vi "G Cluster to PLC Byte Stream.vi"(6 "Byte Length":i32, 8 "error in (no error)":errorcluster, 9 "[Sub-Item Type Descriptor]":T1[](array[typedef]), 10 "Value":variant, 11 "TwinCAT ADS in":refnum<class "TwinCAT ADS.lvclass">) -> (0 "error out":errorcluster, 2 "Byte Stream":u8[](array[numeric]), 3 "TwinCAT ADS out":refnum<class "TwinCAT ADS.lvclass">)   [LabVIEW 2018, in "TwinCAT ADS.lvclass"]
uses:
  TwinCAT ADS.lvclass
  Controls/PLC Sub-Item Type Descriptor.ctl
  Controls/PLC Type.ctl
  G Primitive to PLC Byte Stream.vi/ebfc1059-5ad7-41af-9a32-6ba056cec1e2.vi
  G Primitive to PLC Byte Stream.vi/6e01a951-886b-41b5-8cd1-fdd71fd1a533.vi
  G Primitive to PLC Byte Stream.vi/09c7a0ef-3209-4624-b801-f77696e71225.vi
  G Primitive to PLC Byte Stream.vi/97b8602c-6a72-408e-90bf-08a26de32539.vi
  G Primitive to PLC Byte Stream.vi/0fd4fbf3-4a18-432c-8f70-6a5c8fef8454.vi
  G Primitive to PLC Byte Stream.vi/afdb5a5e-237c-4be5-828e-15f510cf6cea.vi
  G Primitive to PLC Byte Stream.vi/185a6e12-4d7d-4ad7-9936-0525adb2f85e.vi
  G Primitive to PLC Byte Stream.vi/88229fb8-b58c-494b-bd2b-fea6e0d0ed1b.vi
  G Primitive to PLC Byte Stream.vi/e57df404-389c-41d0-a67c-37c75754ab31.vi
  G Primitive to PLC Byte Stream.vi/d0ee652c-9b86-46ed-9065-57d03aa8de3e.vi
  G Primitive to PLC Byte Stream.vi/886bf0b9-f01c-4a44-b2e2-abccc7b97bfa.vi
  G Primitive to PLC Byte Stream.vi/35f71df7-fc14-4c4d-983c-cf72c138dc9e.vi
  G Primitive to PLC Byte Stream.vi/2d2bc992-a9ff-4dd8-b8fe-74c21cb85899.vi
  G Primitive to PLC Byte Stream.vi/100e4a11-5e4a-45b7-be98-adc9eaebd48d.vi
  G Primitive to PLC Byte Stream.vi/132946d9-68c7-4ade-a66d-dc369520c644.vi
  <vilib>/Utility/error.llb/Trim Whitespace.vi
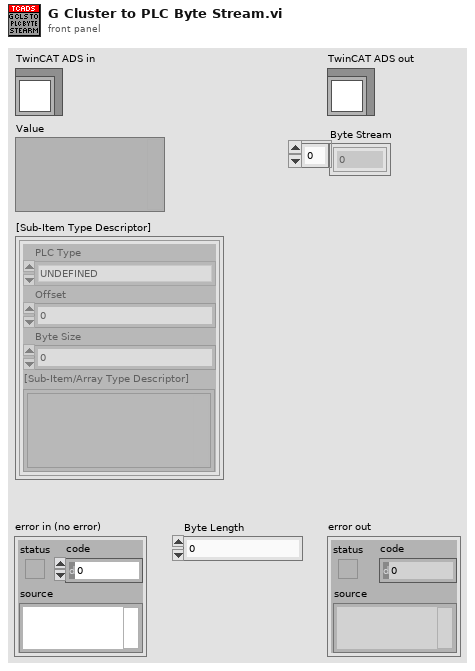
[diagram p1: front panel]
types:
  T1 = typedef "TwinCAT ADS.lvclass/PLC Sub-Item Type Descriptor.ctl" = cluster{"PLC Type":T2, "Offset":i32, "Byte Size":i32, "[Sub-Item/Array Type Descriptor]":variant[]}
  T2 = typedef "TwinCAT ADS.lvclass/PLC Type.ctl" = enum16{"UNDEFINED", "INT", "DINT", "REAL", "LREAL", "SINT", "BYTE", "UINT", "UDINT", "LINT", "ULINT", "STRING", "WSTRING", "BOOL", "TIME", "LTIME", "DATE", "DT", "TOD", "ARRAY", "JAGGED ARRAY", "STRUCT", "FUNCTION BLOCK", "UNION", "POINTER", "USER DEFINED"}
  T3 = typedef "TwinCAT ADS.lvclass/PLC Array Type Descriptor.ctl" = cluster{"Fundamental PLC Type":T2, "Fundamental Type Byte Size":i32, "Item Count":i32, "Dimension Lengths":i32[], "Sub-Item Type Descriptor":variant}
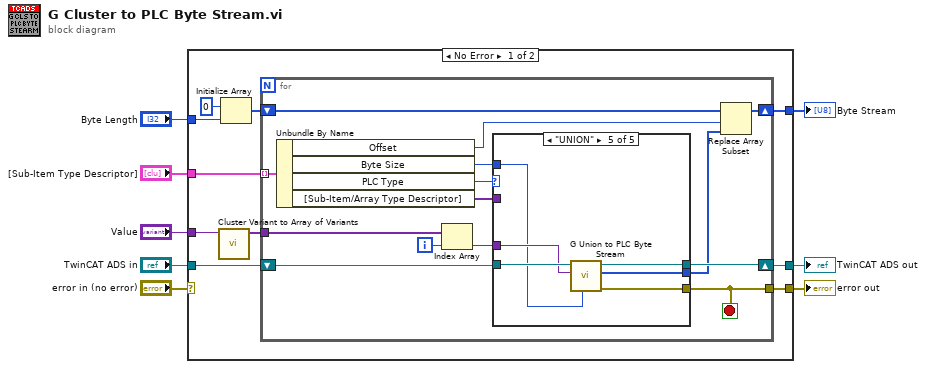
[diagram p0: block diagram]
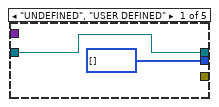
[diagram p2: hidden frame]
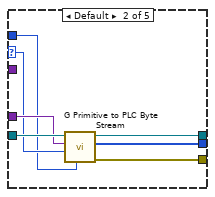
[diagram p3: hidden frame]
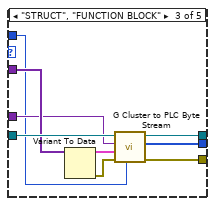
[diagram p4: hidden frame]
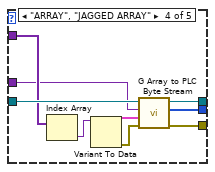
[diagram p5: hidden frame]
diagram:
  n1 = case shown="No Error" "error in (no error)" {
    selector: "error in (no error)" -> [_ w66]
    tunnel: "TwinCAT ADS in" -> [w18 w67]
    tunnel: [w17 w67] -> w7
    tunnel: "[Sub-Item Type Descriptor]" -> [w16 _]
    tunnel: "Value" -> [w15 _]
    tunnel: "Byte Length" -> [w14 _]
    tunnel: [w13 w66] -> w3
    tunnel: [w12 _] -> w2
    frame No Error {
      n2 = call "Cluster Variant to Array of Variants.vi"("Cluster Variant"=w15) -> ("[Variant]"=w11:variant[])  [unwired: 9 in, 1 out]
      n3 = Initialize Array(u8 0 ("Offset"), w14) -> (w9:u8[])
      n4 = for {
        shift-right: [w31] -> w17
        shift-left: w18 -> [w32]
        tunnel: w16 -> [w30] mode=indexing
        tunnel: w11 -> [w29]
        shift-right: [w23] -> w12
        shift-left: w9 -> [w24]
        tunnel: [w27] -> w13
        i -> [w28]
        stop <- w27 stop-if-true
        n5 = Unbundle By Name(w30) -> ("Offset"=w20:i32, "Byte Size"=w21:i32, "PLC Type"=w26:T2, "[Sub-Item/Array Type Descriptor]"=w25:variant[])
        n6 = Index Array(array=w29, index=w28) -> (element=w19:variant)
        n7 = case shown="\"UNION\"" w26 {
          selector: w26 -> [_ w37 _ _ _]
          tunnel: w32 -> [w34 w41 w50 w59 w65]
          tunnel: [w34 w39 w49 w52 w63] -> w31
          tunnel: [_ w40 w48 w53 w64] -> w27
          tunnel: w25 -> [_ _ w47 w58 _]
          tunnel: w19 -> [_ w38 w44 w56 w61]
          tunnel: [u8[] [] ("initialized array") w36 w43 w51 w62] -> w22
          tunnel: w21 -> [_ w35 w42 _ w60]
          frame "UNDEFINED", "USER DEFINED" {
          }
          frame Default {
            n8 = call "G Primitive to PLC Byte Stream.vi"("Byte Length"=w35, "PLC Type"=w37, "Value"=w38, "TwinCAT ADS in"=w41) -> ("error out"=w40:errorcluster, "Byte Stream"=w36:u8[], "TwinCAT ADS out"=w39:refnum<class "TwinCAT ADS.lvclass">)  [unwired: 5 in]
          }
          frame "STRUCT", "FUNCTION BLOCK" {
            n9 = Variant To Data(Variant=w47) -> (data=w45:T1[], error out=w46:errorcluster)  [unwired: 2 in]
            n10 = call "G Cluster to PLC Byte Stream.vi"("Byte Length"=w42, "error in (no error)"=w46, "[Sub-Item Type Descriptor]"=w45, "Value"=w44, "TwinCAT ADS in"=w50) -> ("error out"=w48:errorcluster, "Byte Stream"=w43:u8[], "TwinCAT ADS out"=w49:refnum<class "TwinCAT ADS.lvclass">)  [unwired: 4 in]
          }
          frame "ARRAY", "JAGGED ARRAY" {
            n11 = Index Array(array=w58) -> (element=w57:variant)  [unwired: 1 in]
            n12 = Variant To Data(Variant=w57) -> (data=w54:T3, error out=w55:errorcluster)  [unwired: 2 in]
            n13 = call "G Array to PLC Byte Stream.vi"("error in (no error)"=w55, "Array Information"=w54, "Value"=w56, "TwinCAT ADS in"=w59) -> ("error out"=w53:errorcluster, "Byte Stream"=w51:u8[], "TwinCAT ADS out"=w52:refnum<class "TwinCAT ADS.lvclass">)  [unwired: 5 in]
          }
          frame "UNION" {
            n14 = call "G Union to PLC Byte Stream.vi"("Byte Length"=w60, "Value"=w61, "TwinCAT ADS in"=w65) -> ("error out"=w64:errorcluster, "Byte Stream"=w62:u8[], "TwinCAT ADS out"=w63:refnum<class "TwinCAT ADS.lvclass">)  [unwired: 6 in]
          }
        }
        n15 = Replace Array Subset(array=w24, new element=w22, index=w20) -> (w23:u8[])
      }
    }
    frame Error {
    }
  }
  "error out" <- w3
  "TwinCAT ADS out" <- w7
  "Byte Stream" <- w2
